vi "FTW-Example-Service-Connect.vi"(0 "IP Address":string, 9 "Timeout":i32=1000 format="%dmsec", 11 "error in":errorcluster) -> (4 "FTW Actor Connector":refnum<class "FTW-Example-Service.lvclass">, 6 "Subscription Registration Refnum":refnum<event-registration>, 15 "error out":errorcluster)   [LabVIEW 2013, in "FTW-Example-Service.lvclass"]
uses:
  FTW-Example-Service.lvclass
  source/actor/Message/Base/FTW-Message.lvclass
  FTW-Example-Service.lvclass/FTW-Example-Service.ctl
  source/actor/Subscriber/FTW-Subscriber.lvclass
panel:
  in  "Number":u32
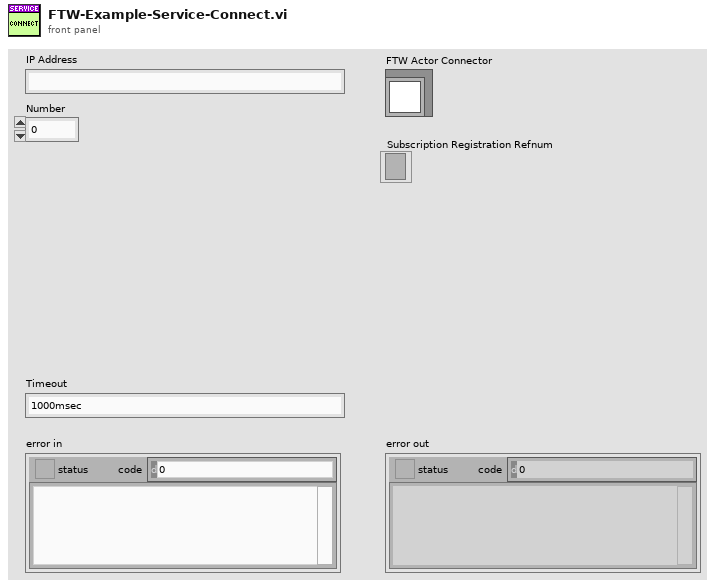
[diagram p1: front panel]
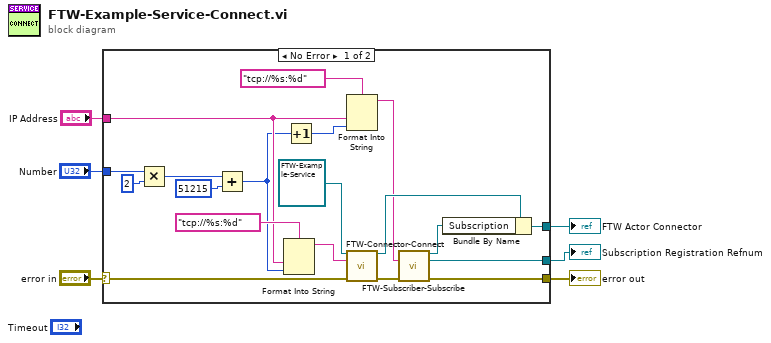
[diagram p0: block diagram]
diagram:
  n1 = case shown="No Error" "error in" {
    selector: "error in" -> [w22 w26]
    tunnel: "IP Address" -> [w18 _]
    tunnel: [w17 _] -> w4
    tunnel: [w16 w26] -> w3
    tunnel: [w13 _] -> w2
    tunnel: "Number" -> [w9 _]
    frame No Error {
      n2 = Multiply(x=w9, y=u32 2) -> (x*y=w11:u32)
      n3 = Add(x=w11, y=u32 51215) -> (x+y=w8:u32)
      n4 = Format Into String(format string="tcp://%s:%d" ("Configuration"), w18, w8) -> (resulting string=w20:string)  [unwired: 2 in, 1 out]
      n5 = Increment(x=w8) -> (x+1=w7:u32)
      n6 = Format Into String(format string="tcp://%s:%d" ("Configuration"), w18, w7) -> (resulting string=w15:string)  [unwired: 2 in, 1 out]
      n7 = call-dynamic "FTW-Connector-Connect.vi"("FTW Actor Connector Type"=refnum<class "FTW-Example-Service.lvclass"> refnum ("TTK_Splashscreen.lvclass"), "Instance Inbox Address"=w20, "error in"=w22) -> ("FTW Actor Connector"=w23:refnum<class "FTW-Example-Service.lvclass">, "error out"=w24:errorcluster)  [unwired: 11 in]
      n8 = call "FTW-Subscriber-Subscribe.vi"("Addresses"=w15, "error in"=w24) -> ("FTW-Subscription Out"=w14:refnum<class "FTW-Subscriber.lvclass">, "Subscriber Registration"=w13:refnum<event-registration>, "error out"=w16:errorcluster)  [unwired: 11 in]
      n9 = Bundle By Name(cluster=w23, "Subscription"=w14) -> (w17:refnum<class "FTW-Example-Service.lvclass">)
    }
    frame Error {
    }
  }
  "error out" <- w3
  "FTW Actor Connector" <- w4
  "Subscription Registration Refnum" <- w2
